vi "CalcChannelWidth.vi"(1 "TAC gain":u16, 2 "channel count":i32, 3 "TAC window (ns)":dbl format="%.2f") -> (0 "channel width (ns)":dbl format="%.2f")   [LabVIEW 2009]
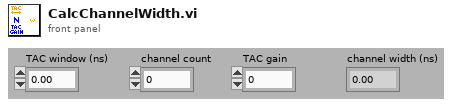
[diagram p1: front panel]
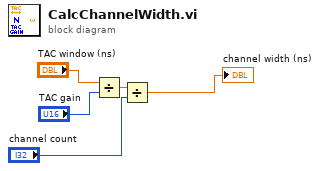
[diagram p0: block diagram]
diagram:
  n1 = Divide(x="TAC window (ns)", y="TAC gain") -> (x/y=w3:dbl)
  n2 = Divide(x=w3, y="channel count") -> (x/y=→"channel width (ns)":dbl)
